vi "AddData.vi"() -> (2 "?":bool, 3 "ProgramData 2":T1={"Numer Produktu"="abc", "Nazwa Produktu"="dd", "Wytwórca"="ss"})   [LabVIEW 2019]
uses:
  ProductsCluster.ctl
panel:
  in  "ProgramData":T1
  in  "Cancel Button":bool
  in  "OK Button":bool
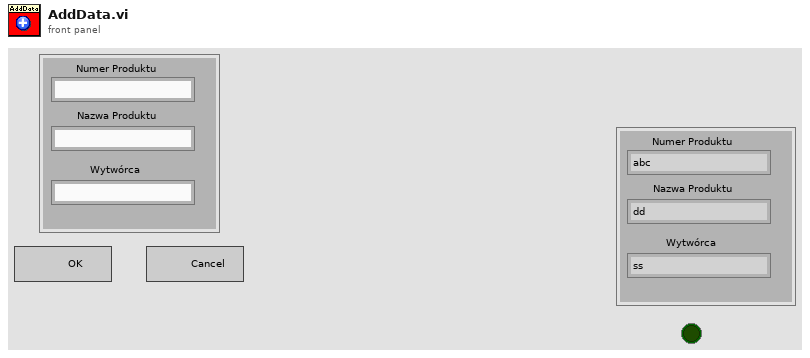
[diagram p1: front panel]
types:
  T1 = typedef "ProductsCluster.ctl" = cluster{"Numer Produktu":string, "Nazwa Produktu":string, "Wytwórca":string}
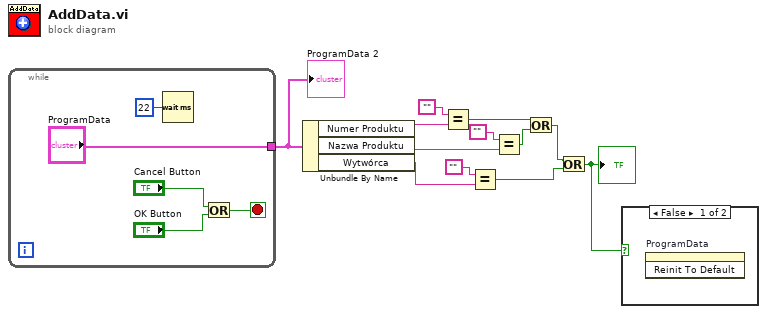
[diagram p0: block diagram]
diagram:
  n1 = while {
    tunnel: ["ProgramData"] -> w2
    stop <- w16 stop-if-true
    n2 = Wait (ms)(milliseconds to wait=u32 22) -> ()  [unwired: 1 out]
    n3 = Or(x="Cancel Button", y="OK Button") -> (x .or. y?=w16:bool)
  }
  "ProgramData 2" <- w2
  n4 = Unbundle By Name(w2) -> ("Numer Produktu"=w12:string, "Nazwa Produktu"=w9:string, "Wytwórca"=w7:string)
  n5 = Equal?(x="", y=w12) -> (x = y?=w6:bool)
  n6 = Equal?(x="", y=w7) -> (x = y?=w3:bool)
  n7 = Equal?(x="", y=w9) -> (x = y?=w5:bool)
  n8 = Or(x=w6, y=w5) -> (x .or. y?=w4:bool)
  n9 = Or(x=w4, y=w3) -> (x .or. y?=w1:bool)
  "?" <- w1
  n10 = case shown="False" w1 {
    frame False {
      n11 = invoke on="ProgramData" class="Clust (strict)" method="Reinit To Default"() -> ()  [unwired: 3 in, 3 out]
    }
    frame True {
    }
  }
